vi "gfitsio-write-key-datetime.vi"(6 "comment":string, 7 "keyname":string, 8 "error in (no error)":errorcluster, 9 "value":timestamp, 11 "gfits refnum":T1) -> (0 "error out":errorcluster, 3 "dup gfits refnum":T1)   [LabVIEW 2024, in "gfitsio.lvlib"]
doc: "Write a keyword of the appropriate data type into the current HDU. If the keyword already exists it will be overwritten. Otherwise a new keyword will be appended to the header."
uses:
  gfitsio.lvlib
  gfitsio-refnum.ctl
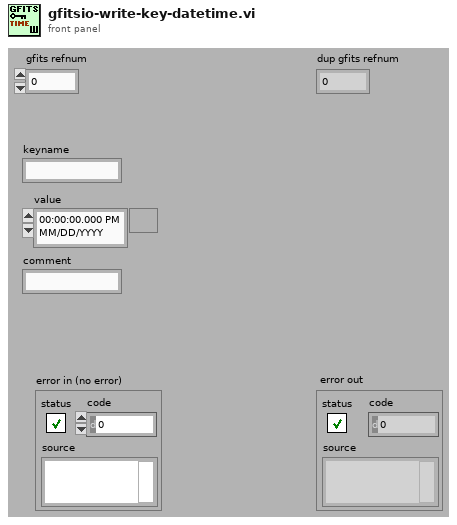
[diagram p1: front panel]
types:
  T1 = typedef "gfitsio.lvlib/gfitsio-refnum.ctl" = u64
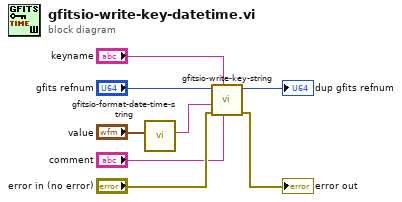
[diagram p0: block diagram]
diagram:
  n1 = call "gfitsio-format-date-time-string.vi"("timestamp"="value") -> ("date/time string"=w3:string)  [unwired: 10 out]
  n2 = call "gfitsio-write-key-string.vi"("comment"="comment", "keyname"="keyname", "error in (no error)"="error in (no error)", "value"=w3, "gfits refnum"="gfits refnum") -> ("error out"=→"error out":errorcluster, "dup gfits refnum"=→"dup gfits refnum":T1)  [unwired: 1 in, 4 out]
